vi "_CH_LM Default Instrument Setup.vi"(0 "Meter Index":i32, 5 "error in (no error)":errorcluster, 7 "Timeout / ms (3000)":i32=3000, 9 "Lock Timeout / ms (1000)":i32=1000) -> (11 "Lock timed out":bool, 14 "Meter Index":i32, 19 "error out":errorcluster)   [LabVIEW 2012, in "CH_LM.lvlib"]
doc: "This Utility VI sends a default command string to the instrument whenever a new session is opened, or the instrument is reset. Use this VI as a subVI for the Initialize and Reset VIs. Altering this VI could cause these two VIs to operate incorrectly.\n\n<B>Attention:</B> You should not delete or modify the first two subVIs.\n1. An instrument should be set to remote mode to avoid concurrent local and remote operation.\n2. Do not change the array with Data Tokens. They are requiered as set. Otherwise the CH_LM Measurement Fetch Data.vi will not work properly."
uses:
  CH_LM.lvlib
  CH_LM/CH_LM Data Token.ctl
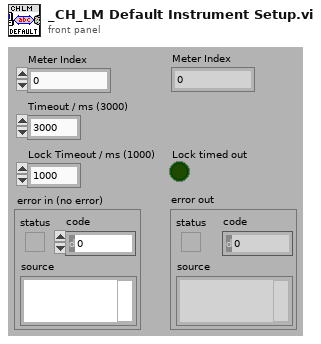
[diagram p1: front panel]
types:
  T1 = typedef "CH_LM.lvlib/CH_LM Data Token.ctl" = enum16{"Raw data", "Quad distance", "Formated data", "Unit", "Pulse period", "Flags", "Sequence ID"}
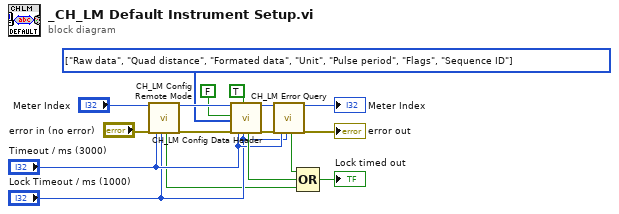
[diagram p0: block diagram]
diagram:
  w3 = T1[] [enum."Raw data", enum."Quad distance", enum."Formated data", enum."Unit", enum."Pulse period", enum."Flags", enum."Sequence ID"] items=["Raw data", "Quad distance", "Formated data", "Unit", "Pulse period", "Flags", "Sequence ID"] ("Data Tokens")
  n1 = call "CH_LM Config Remote Mode.vi"("Meter Index"="Meter Index", "error in (no error)"="error in (no error)", "Timeout / ms (3000)"="Timeout / ms (3000)", "Lock Timeout / ms (1000)"="Lock Timeout / ms (1000)") -> ("Lock timed out"=w8:bool, "Meter Index"=w12:i32, "error out"=w11:errorcluster)  [unwired: 13 out]
  n2 = call "CH_LM Config Data Header.vi"("Meter Index"=w12, "Data Header (disable)"=FALSE, "Data Tokens"=w3, "error in (no error)"=w11, "Timeout / ms (3000)"="Timeout / ms (3000)", "Action (query)"=TRUE, "Lock Timeout / ms (1000)"="Lock Timeout / ms (1000)") -> ("Lock timed out"=w13:bool, "Meter Index"=w2:i32, "error out"=w1:errorcluster)  [unwired: 10 out]
  n3 = call "CH_LM Error Query.vi"("Meter Index"=w2, "error in (no error)"=w1, "Timeout / ms (3000)"="Timeout / ms (3000)", "Lock Timeout / ms (1000)"="Lock Timeout / ms (1000)") -> ("Lock timed out"=w15:bool, "Meter Index"=→"Meter Index":i32, "error out"=→"error out":errorcluster)  [unwired: 13 out]
  n4 = Compound Arithmetic op=OR(w15, w13, w8) -> (→"Lock timed out":bool)
